vi "VI-Create Serialized KObject.vi"(0 "Folder":path=path "C:/Users/Ken/Desktop", 2 "Base class path":path=path "C:/Users/Ken/Desktop/Base/Base.lvclass", 7 "Name":string="Class1", 9 "Make base":bool=TRUE, 11 "error in (no error)":errorcluster) -> (4 "Library":path, 15 "error out":errorcluster)   [LabVIEW 2020]
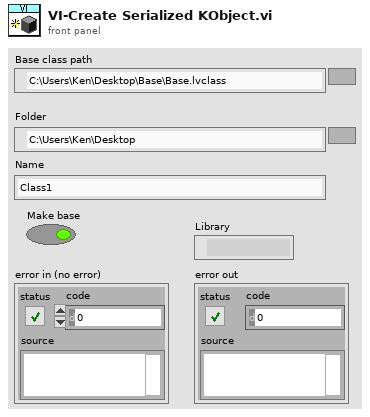
[diagram p1: front panel]
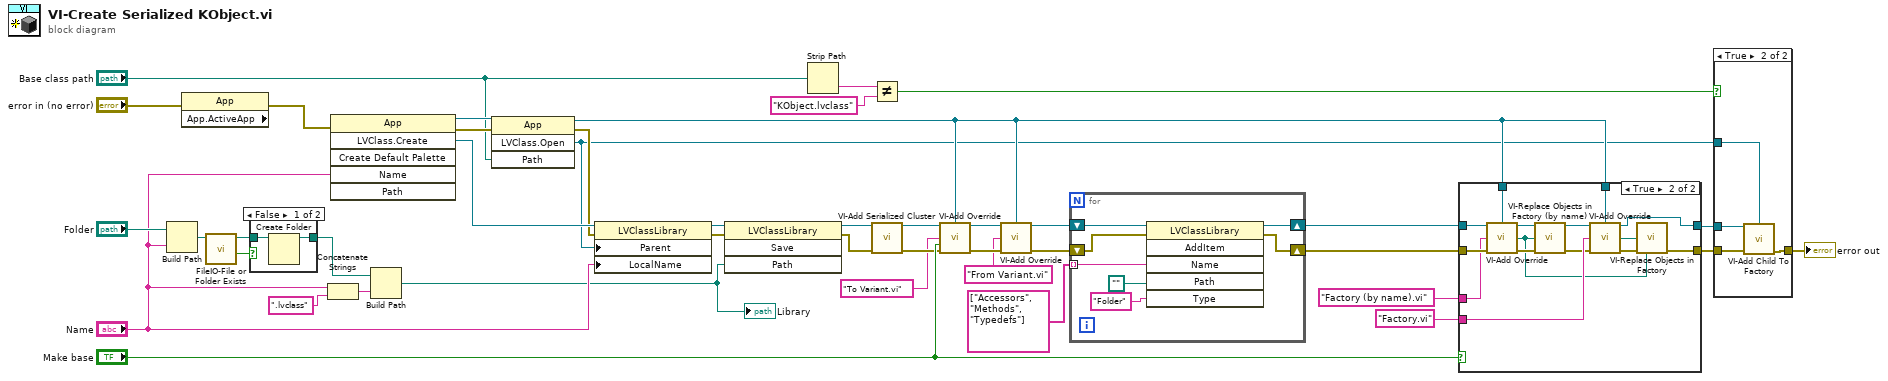
[diagram p0: block diagram]
diagram:
  n1 = Build Path(base path="Folder", name or relative path="Name") -> (appended path=w41:path)
  n2 = property class="App" props=["App.ActiveApp"](error in="error in (no error)") -> (error out=w35:errorcluster)  [unwired: 1 in, 2 out]
  n3 = call "FileIO-File or Folder Exists.vi"("path"=w41) -> ("Exists?"=w39:bool, "dup path"=w40:path)  [unwired: 7 in, 2 out]
  n4 = case shown="False" w39 {
    tunnel: [w44 w45] -> w34
    tunnel: w40 -> [w43 w45]
    frame False {
      n5 = Create Folder(path (use dialog)=w43) -> (created path=w44:path)  [unwired: 2 in, 2 out]
    }
    frame True {
    }
  }
  n6 = Concatenate Strings("Name", ".lvclass" ("string")) -> (w38:string)
  n7 = invoke class="App" method="LVClass.Create"(error in=w35, "Name"="Name") -> (reference out=w30:refnum<vi>, error out=w29:errorcluster, "LVClass.Create"=w33:refnum<vi>)  [unwired: 4 in, 3 out]
  n8 = Build Path(base path=w34, name or relative path=w38) -> (appended path=w15:path)
  "Library" <- w15
  n9 = invoke class="App" method="LVClass.Open"(reference=w30, error in=w29, "Path"="Base class path") -> (reference out=w25:refnum<vi>, error out=w28:errorcluster, "LVClass.Open"=w12:refnum<vi>)  [unwired: 1 in, 1 out]
  n10 = property class="LVClassLibrary"(reference=w33, error in=w28, "Parent"=w12, "LocalName"="Name") -> (reference out=w32:refnum<vi>, error out=w31:errorcluster)
  n11 = invoke class="LVClassLibrary" method="Save"(reference=w32, error in=w31, "Path"=w15) -> (reference out=w6:refnum<vi>, error out=w24:errorcluster)  [unwired: 1 in, 2 out]
  n12 = Strip Path(path="Base class path") -> (name=w9:string)  [unwired: 1 out]
  n13 = Not Equal?(x=w9, y="KObject.lvclass") -> (x != y?=w7:bool)
  n14 = call "VI-Add Serialized Cluster.vi"("LVClass.Create in"=w6, "error in (no error)"=w24) -> ("LVClassLibrary out"=w21:refnum<vi>, "error out"=w23:errorcluster)  [unwired: 12 in]
  n15 = call "VI-Add Override.vi"("LVClassLibrary in"=w21, "application refnum"=w25, "Method"="To Variant.vi" ("name or relative path"), "Base class"="Make base", "error in (no error)"=w23) -> ("reference out"=w16:refnum<vi>, "error out"=w20:errorcluster)  [unwired: 8 in, 1 out]
  n16 = call "VI-Add Override.vi"("LVClassLibrary in"=w16, "application refnum"=w25, "Method"="From Variant.vi" ("name or relative path"), "error in (no error)"=w20) -> ("reference out"=w3:refnum<vi>, "error out"=w4:errorcluster)  [unwired: 9 in, 1 out]
  n17 = for {
    shift-right: [w52] -> w5
    shift-left: w4 -> [w51]
    shift-right: [w47] -> w2
    shift-left: w3 -> [w50]
    tunnel: string[] ["Accessors", "Methods", "Typedefs"] ("Name") -> [w46] mode=indexing
    n18 = invoke class="LVClassLibrary" method="AddItem"(reference=w50, error in=w51, "Name"=w46, "Path"=path "", "Type"="Folder" ("Name")) -> (reference out=w47:refnum<vi>, error out=w52:errorcluster)  [unwired: 1 in, 4 out]
  }
  n19 = case shown="True" "Make base" {
    tunnel: w5 -> [w54 w69]
    tunnel: [w53 w57] -> w13
    tunnel: [w54 w56] -> w14
    tunnel: "Factory (by name).vi" ("name or relative path") -> [_ w68]
    tunnel: "Factory.vi" ("name or relative path") -> [_ w67]
    tunnel: w25 -> [_ w59]
    tunnel: w25 -> [_ w58]
    tunnel: w2 -> [w53 w55]
    frame False {
    }
    frame True {
      n20 = call "VI-Add Override.vi"("LVClassLibrary in"=w55, "application refnum"=w59, "Method"=w68, "error in (no error)"=w69) -> ("reference out"=w61:refnum<vi>, "file path"=w62:path, "error out"=w66:errorcluster)  [unwired: 9 in]
      n21 = call "VI-Replace Objects in Factory (by name).vi"("LVClassLibrary in"=w61, "vi path"=w62, "error in (no error)"=w66) -> ("reference out"=w60:refnum<vi>, "error out"=w65:errorcluster)  [unwired: 11 in]
      n22 = call "VI-Add Override.vi"("LVClassLibrary in"=w60, "application refnum"=w58, "Method"=w67, "error in (no error)"=w65) -> ("reference out"=w57:refnum<vi>, "file path"=w63:path, "error out"=w64:errorcluster)  [unwired: 9 in]
      n23 = call "VI-Replace Objects in Factory.vi"("vi path"=w63, "error in (no error)"=w64, "by name"=w62) -> ("error out"=w56:errorcluster)  [unwired: 12 in]
    }
  }
  n24 = case shown="True" w7 {
    tunnel: w14 -> [w70 w74]
    tunnel: w13 -> [_ w73]
    tunnel: w12 -> [_ w72]
    tunnel: [w70 w71] -> w11
    frame False {
    }
    frame True {
      n25 = call "VI-Add Child To Factory.vi"("LVClassLibrary in"=w73, "Parent"=w72, "error in (no error)"=w74) -> ("error out"=w71:errorcluster)  [unwired: 11 in, 1 out]
    }
  }
  "error out" <- w11
